vi "init_laser_power_Q.vi"(2 "max queue size (-1, unlimited)":i32) -> (8 "Laser Power Q":T1)   [LabVIEW 2023]
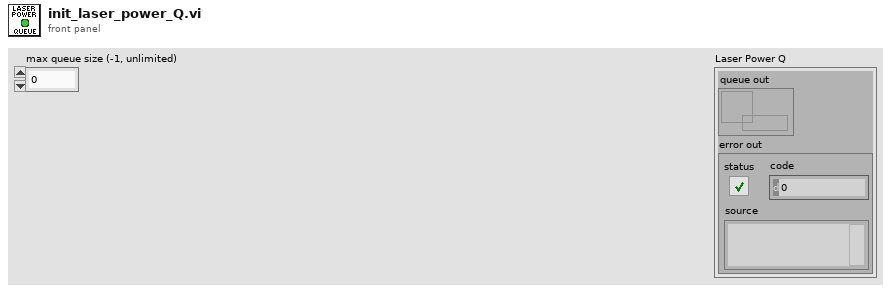
[diagram p1: front panel]
types:
  T1 = cluster{"queue out":refnum<queue>, "error out":errorcluster}
  T2 = cluster{"Power Reading ":dbl, "T imestamp":dbl, "Status":i32}
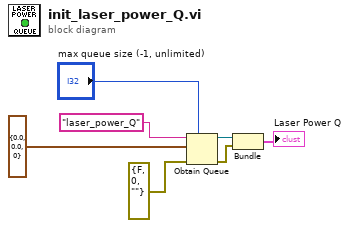
[diagram p0: block diagram]
diagram:
  n1 = Obtain Queue(max queue size (-1, unlimited)="max queue size (-1, unlimited)", name (unnamed)="laser_power_Q", element data type=T2 {"Power Reading "=0.0, "T imestamp"=0.0, "Status"=0}, error in (no error)=errorcluster {"status"=FALSE, "code"=0, "source"=""}) -> (queue out=w7:refnum<queue>, error out=w6:errorcluster)  [unwired: 1 in, 1 out]
  n2 = Bundle("queue out"=w7, "error out"=w6) -> (→"Laser Power Q":T1)  [unwired: 1 in]
